vi "StopICL.vi"(8 "error in (no error)":errorcluster, 11 "DeviceManager in":refnum<class "DeviceManager.lvclass">) -> (0 "error out":errorcluster, 3 "DeviceManager out":refnum<class "DeviceManager.lvclass">)   [LabVIEW 2023, in "DeviceManager.lvclass"]
uses:
  DeviceManager.lvclass
  DeviceManager.lvclass/DeviceManager.ctl
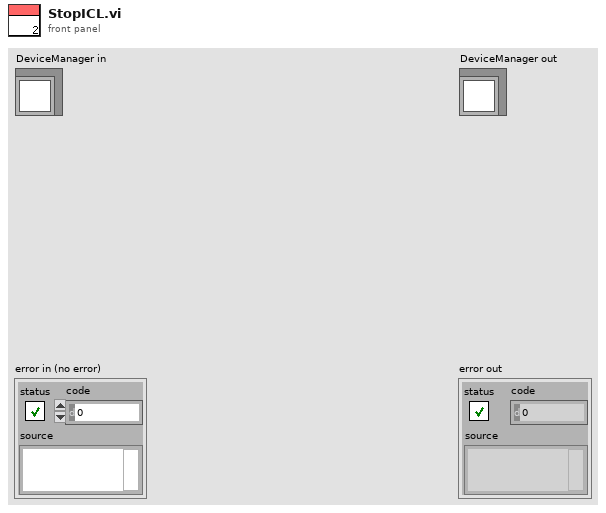
[diagram p1: front panel]
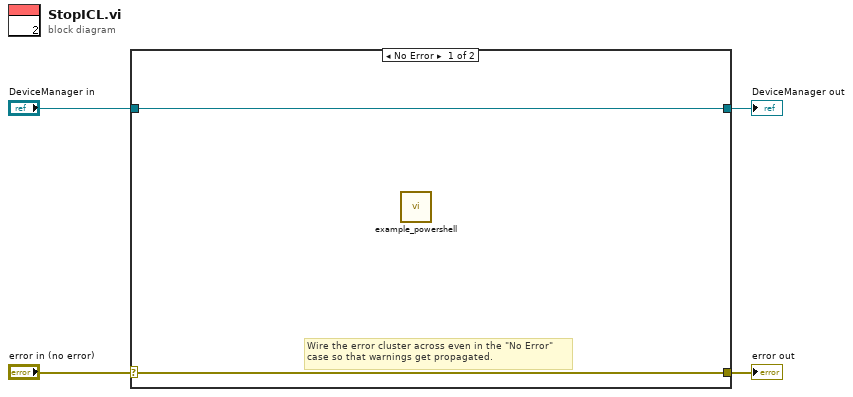
[diagram p0: block diagram]
diagram:
  n1 = case shown="No Error" "error in (no error)" {
    selector: "error in (no error)" -> [w5 w8]
    tunnel: [w5 w8] -> w3
    tunnel: [w6 w7] -> w1
    tunnel: "DeviceManager in" -> [w6 w7]
    frame No Error {
      # "Wire the error cluster across even in the \"No Error\"\ncase so that warnings get propagated."
      n2 = call <vilib>:"example_powershell.vi"() -> ()  [unwired: 12 in]
    }
    frame Error {
    }
  }
  "error out" <- w3
  "DeviceManager out" <- w1
